vi "Inline - Update Error Counters Channels.vi"(6 "Inline Status Channels Refs":T1[](array[typedef]) format="%.0x", 8 "error in (no error)":errorcluster, 11 "msgact":u8) -> (0 "error IO":errorcluster, 1 "Bit Error":bool, 3 "Hit":bool)   [LabVIEW 2016, in "Ballard Arinc-429 Engine.lvlib"]
uses:
  Ballard Arinc-429 Engine.lvlib
  <vilib>/NI Veristand/Custom Device API/Data Reference.ctl
  <vilib>/NI VeriStand/Custom Device Tools/Custom Device Utility Library/Custom Device Utility Library.lvlib
  <vilib>/NI VeriStand/Custom Device API/Custom Device API.lvlib
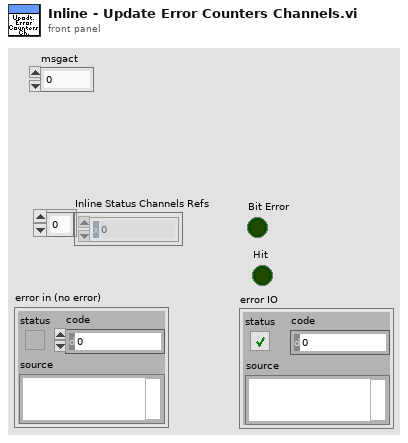
[diagram p1: front panel]
types:
  T1 = typedef "Custom Device API.lvlib/Data Reference.ctl" = i32
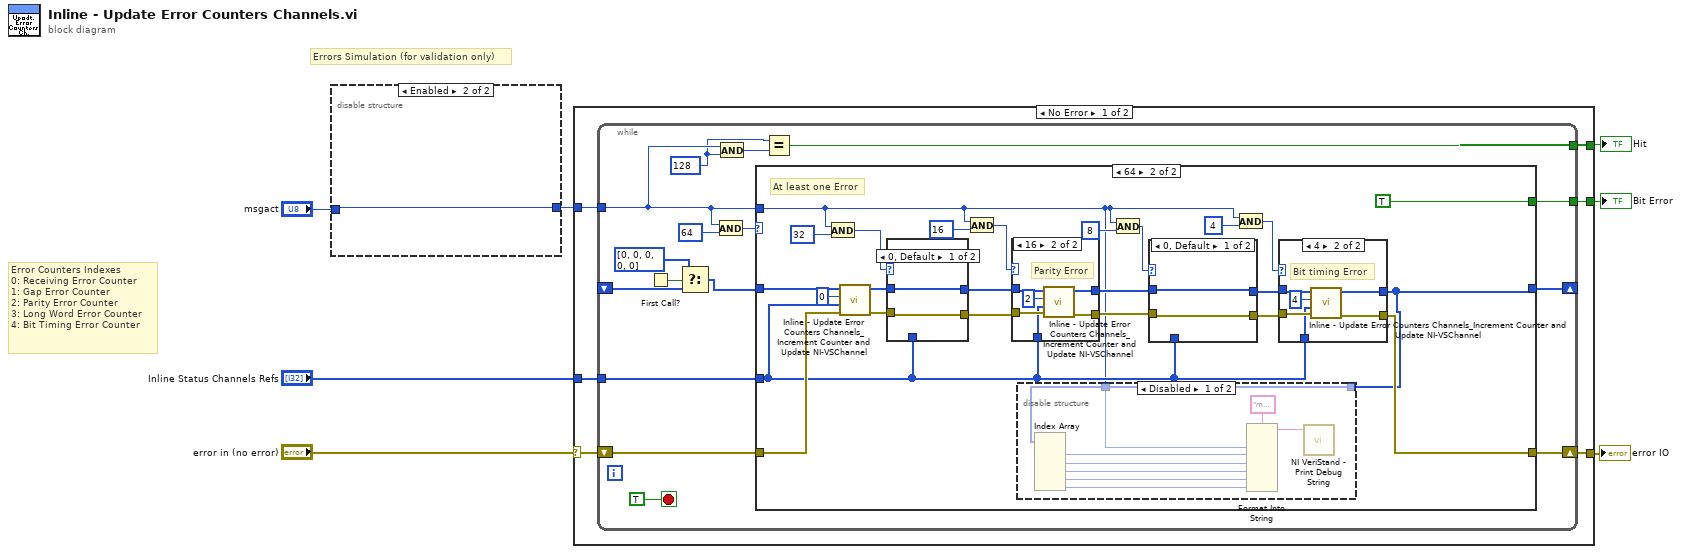
[diagram p0: block diagram]
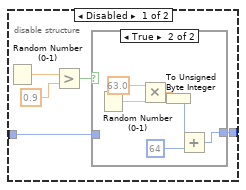
[diagram p2: hidden frame]
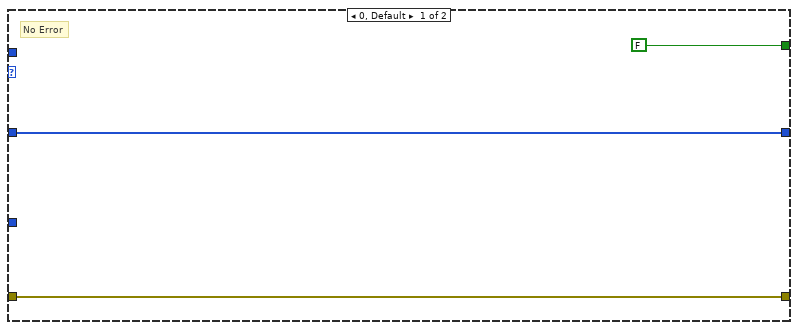
[diagram p4: hidden frame]
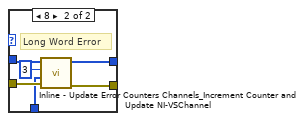
[diagram p7: hidden frame]
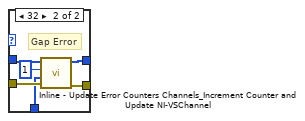
[diagram p9: hidden frame]
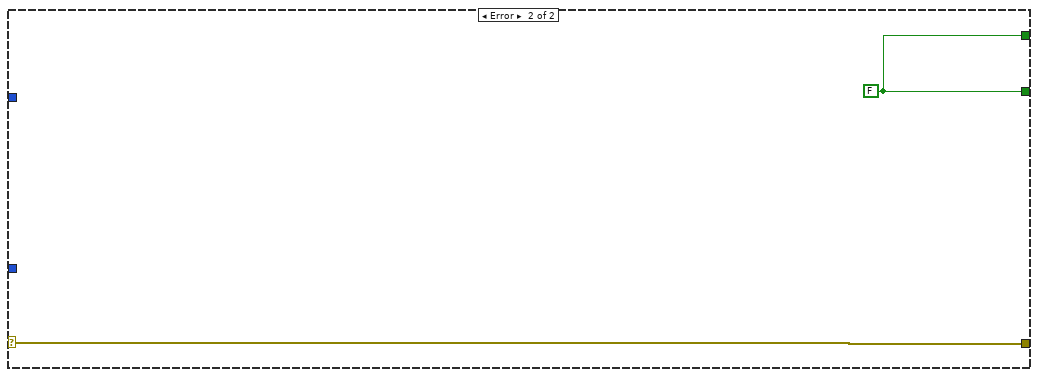
[diagram p10: hidden frame]
diagram:
  # "Errors Simulation (for validation only)"
  # "Error Counters Indexes\n0: Receiving Error Counter\n1: Gap Error Counter\n2: Parity Error Counter\n3: Long Word Error Counter\n4: Bit Timing Error Counter"
  n1 = disable-structure shown="Enabled" {
    disable-tunnel: "msgact" -> [w9 w20]
    disable-tunnel: [w8 w20] -> w1
    frame Disabled {
      n2 = Random Number (0-1)() -> (number: 0 to 1=w12:dbl)
      n3 = Greater?(x=w12, y=0.9) -> (0:w10:bool)
      n4 = case shown="True" w10 {
        tunnel: w9 -> [w13 _]
        tunnel: [w13 w18] -> w8
        frame False {
        }
        frame True {
          n5 = Random Number (0-1)() -> (number: 0 to 1=w17:dbl)
          n6 = Multiply(x=63.0, y=w17) -> (x*y=w15:dbl)
          n7 = To Unsigned Byte Integer(number=w15) -> (unsigned 8bit integer=w14:u8)
          n8 = Add(x=w14, y=u8 64) -> (x+y=w18:u8)
        }
      }
    }
    frame Enabled {
    }
  }
  n9 = case shown="No Error" "error in (no error)" {
    selector: "error in (no error)" -> [w24 w112]
    tunnel: "Inline Status Channels Refs" -> [w26 _]
    tunnel: w1 -> [w25 _]
    tunnel: [w23 w112] -> w5
    tunnel: [w22 w111] -> w4
    tunnel: [w21 w111] -> w3
    frame No Error {
      n10 = while {
        tunnel: w26 -> [w40]
        tunnel: w25 -> [w30]
        shift-right: [w38] -> w23
        shift-left: w24 -> [w39]
        shift-right: [w33] -> _
        shift-left: _ -> [w32]
        tunnel: [w31] -> w22
        tunnel: [w27] -> w21
        stop <- TRUE stop-if-true
        w28 = u8 128 ("y")
        n11 = First Call?() -> (First Call?: T/F=w36:bool)
        n12 = Select(t=u32[] [0, 0, 0, 0, 0], s=w36, f=w32) -> (s? t:f=w35:u32[])
        n13 = And(x=w30, y=u8 64) -> (x .and. y?=w42:u8)
        n14 = And(x=w30, y=w28) -> (x .and. y?=w29:u8)
        n15 = case shown="64" w42 {
          tunnel: w35 -> [w45 w69]
          tunnel: [w45 w46] -> w33
          tunnel: w40 -> [_ w50]
          tunnel: w39 -> [w44 w67]
          tunnel: w30 -> [_ w47]
          tunnel: [w44 w49] -> w38
          tunnel: [FALSE TRUE] -> w31
          frame 0, Default {
            # "No Error"
          }
          frame 64 {
            # "At least one Error"
            n16 = And(x=w47, y=u8 32) -> (x .and. y?=w65:u8)
            n17 = call "Inline - Update Error Counters Channels_Increment Counter and Update NI-VSChannel.vi"("error in (no error)"=w67, "Inline Status Channels Refs"=w50, "index"=0, "Error Counters Value In in"=w69) -> ("error out"=w63:errorcluster, "Error Counters Value In out"=w64:u32[])  [unwired: 6 in]
            n18 = case shown="0, Default" w65 {
              tunnel: w64 -> [w104 w109]
              tunnel: w63 -> [w103 w110]
              tunnel: [w104 w108] -> w60
              tunnel: [w103 w107] -> w59
              tunnel: w50 -> [_ w106]
              frame 0, Default {
              }
              frame 32 {
                # "Gap Error"
                n19 = call "Inline - Update Error Counters Channels_Increment Counter and Update NI-VSChannel.vi"("error in (no error)"=w110, "Inline Status Channels Refs"=w106, "index"=1, "Error Counters Value In in"=w109) -> ("error out"=w107:errorcluster, "Error Counters Value In out"=w108:u32[])  [unwired: 6 in]
              }
            }
            n20 = And(x=w47, y=u8 16) -> (x .and. y?=w61:u8)
            n21 = case shown="16" w61 {
              tunnel: w60 -> [w96 w101]
              tunnel: w59 -> [w95 w102]
              tunnel: [w96 w100] -> w57
              tunnel: [w95 w99] -> w56
              tunnel: w50 -> [_ w98]
              frame 0, Default {
              }
              frame 16 {
                # "Parity Error"
                n22 = call "Inline - Update Error Counters Channels_Increment Counter and Update NI-VSChannel.vi"("error in (no error)"=w102, "Inline Status Channels Refs"=w98, "index"=2, "Error Counters Value In in"=w101) -> ("error out"=w99:errorcluster, "Error Counters Value In out"=w100:u32[])  [unwired: 6 in]
              }
            }
            n23 = And(x=w47, y=u8 8) -> (x .and. y?=w55:u8)
            n24 = case shown="0, Default" w55 {
              tunnel: w57 -> [w88 w93]
              tunnel: w56 -> [w87 w94]
              tunnel: [w88 w92] -> w54
              tunnel: [w87 w91] -> w53
              tunnel: w50 -> [_ w90]
              frame 0, Default {
              }
              frame 8 {
                # "Long Word Error"
                n25 = call "Inline - Update Error Counters Channels_Increment Counter and Update NI-VSChannel.vi"("error in (no error)"=w94, "Inline Status Channels Refs"=w90, "index"=3, "Error Counters Value In in"=w93) -> ("error out"=w91:errorcluster, "Error Counters Value In out"=w92:u32[])  [unwired: 6 in]
              }
            }
            n26 = And(x=w47, y=u8 4) -> (x .and. y?=w51:u8)
            n27 = case shown="4" w51 {
              tunnel: w54 -> [w80 w85]
              tunnel: w53 -> [w79 w86]
              tunnel: [w80 w84] -> w46
              tunnel: [w79 w83] -> w49
              tunnel: w50 -> [_ w82]
              frame 0, Default {
              }
              frame 4 {
                # "Bit timing Error"
                n28 = call "Inline - Update Error Counters Channels_Increment Counter and Update NI-VSChannel.vi"("error in (no error)"=w86, "Inline Status Channels Refs"=w82, "index"=4, "Error Counters Value In in"=w85) -> ("error out"=w83:errorcluster, "Error Counters Value In out"=w84:u32[])  [unwired: 6 in]
              }
            }
            n29 = disable-structure shown="Disabled" {
              disable-tunnel: w47 -> [w77 _]
              disable-tunnel: w46 -> [w75 _]
              frame Disabled {
                n30 = Index Array(array=w75) -> (element #1=w74:u32, element #2=w73:u32, element #3=w72:u32, element #4=w71:u32, element #5=w70:u32)  [unwired: 5 in]
                n31 = Format Into String(format string="msgact: %d. 0: %d, 1: %d, 2: %d, 3: %d, 4: %d.\\n", w77, w74, w73, w72, w71, w70) -> (resulting string=w78:string)  [unwired: 2 in, 1 out]
                n32 = call <vilib>:"NI VeriStand - Print Debug String.vi"("Message"=w78) -> ()  [unwired: 10 in, 1 out]
              }
              frame Enabled {
              }
            }
          }
        }
        n33 = Equal?(x=w28, y=w29) -> (x = y?=w27:bool)
      }
    }
    frame Error {
      w111 = FALSE
    }
  }
  "error IO" <- w5
  "Bit Error" <- w4
  "Hit" <- w3
